vi "Host_NetStreams.vi"() -> ()   [LabVIEW 2019]
uses:
  <vilib>/dex/Flush And Wait Empty Condition.ctl
panel:
  out "error out 2":errorcluster
  out "Waveform Graph":dbl[](graph)
  out "size(s)":i32
  out "error out":errorcluster
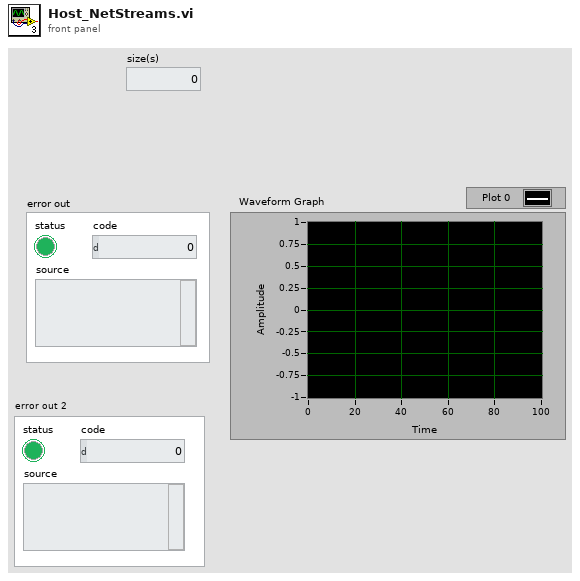
[diagram p1: front panel]
types:
  T1 = typedef "Flush And Wait Empty Condition.ctl" = u8
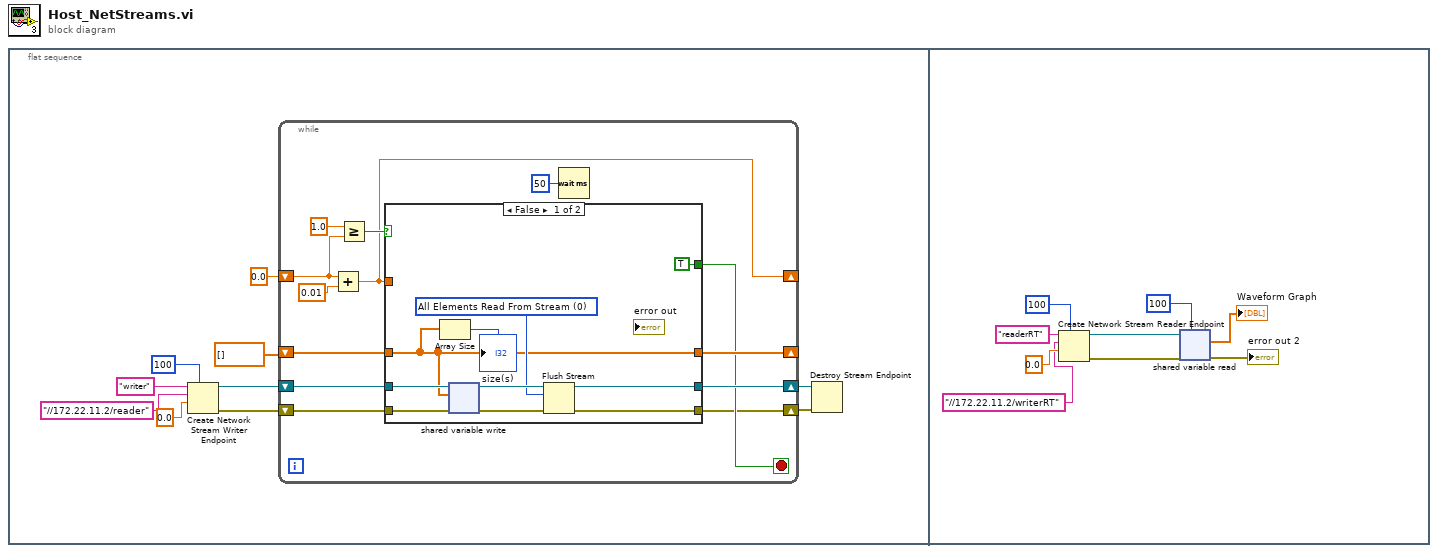
[diagram p0: block diagram]
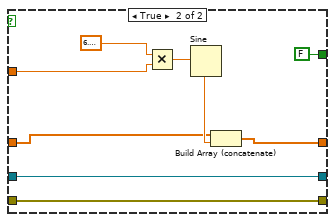
[diagram p2: hidden frame]
diagram:
  n1 = flat-sequence {
    frame #0 {
      n2 = Create Network Stream Writer Endpoint(7:100 ("writer buffer size"), 9:0.0 ("sin(x)"), 10:"//172.22.11.2/reader" ("writer url"), 11:"writer" ("writer name")) -> (0:w7:errorcluster, 3:w8:refnum<k21>)  [unwired: 3 in]
      n3 = while {
        shift-right: [w20] -> w2
        shift-left: w8 -> [w23]
        shift-right: [w11] -> w1
        shift-left: w7 -> [w22]
        shift-right: [w15] -> _
        shift-left: 0.0 ("sin(x)") -> [w18]
        shift-right: [w14] -> _
        shift-left: dbl[] [] -> [w13]
        stop <- w12 stop-if-true
        n4 = Add(x=w18, y=0.01) -> (x+y=w15:dbl)
        n5 = Greater Or Equal?(x=1.0, y=w18) -> (x >= y?=w16:bool)
        n6 = case shown="False" w16 {
          tunnel: w23 -> [w33 w38]
          tunnel: w22 -> [w31 w37]
          tunnel: [w25 w37] -> w11
          tunnel: [w24 w38] -> w20
          tunnel: w15 -> [_ w40]
          tunnel: [w27 w39] -> w14
          tunnel: w13 -> [w27 w34]
          tunnel: [TRUE ("stop") FALSE ("stop")] -> w12
          frame False {
            w28 = T1 0 items=["All Elements Read From Stream", "All Elements Available for Reading"] ("wait condition")
            n7 = Array Size(array=w27) -> (size(s)=→"size(s)":i32)
            n8 = shared-variable-write(w33, w31, w27) -> (w32:refnum<k21>, w30:errorcluster)  [unwired: 1 in, 1 out]
            n9 = Flush Stream(8:w30, 10:w28, 11:w32) -> (0:w25:errorcluster, 3:w24:refnum<k21>)  [unwired: 1 in, 1 out]
          }
          frame True {
            n10 = Multiply(x=6.283185307179586, y=w40) -> (x*y=w42:dbl)
            n11 = Sine(x=w42) -> (sin(x)=w35:dbl)
            n12 = Build Array (concatenate)(w34, w35) -> (w39:dbl[])
          }
        }
        n13 = Wait (ms)(milliseconds to wait=u32 50) -> ()  [unwired: 1 out]
      }
      n14 = Destroy Stream Endpoint(8:w1, 11:w2) -> ()  [unwired: 1 out]
    }
    frame #1 {
      n15 = Create Network Stream Reader Endpoint(7:100 ("reader buffer size"), 9:0.0 ("sin(x)"), 10:"//172.22.11.2/writerRT" ("writer url"), 11:"readerRT" ("reader name")) -> (0:w47:errorcluster, 3:w48:refnum<k21>)  [unwired: 3 in]
      n16 = shared-variable-read(w48, w47, 100 ("# elements")) -> (→"error out 2":errorcluster, →"Waveform Graph":dbl[])  [unwired: 1 in, 2 out]
    }
  }
